vi "A提取产品ID.vi"(10 "字符串":string="B1_011308090450260075.280040.000090.00A000002600000020009999AA ") -> (3 "产品ID":string)   [LabVIEW 2013]
uses:
  <vilib>/Utility/error.llb/whitespace.ctl
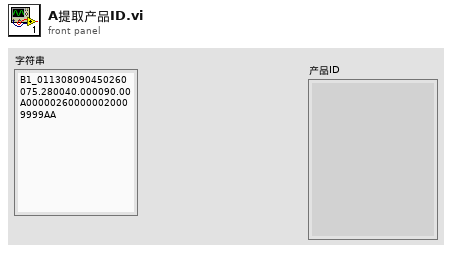
[diagram p1: front panel]
types:
  T1 = typedef "whitespace.ctl" = u16
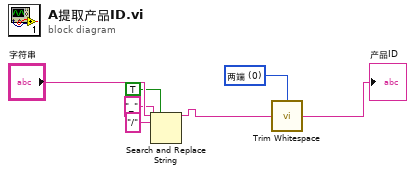
[diagram p0: block diagram]
diagram:
  w1 = T1 0 items=["两端", "字符串首端", "字符串末端"] ("location (both)")
  n1 = Search and Replace String(replace all?=TRUE ("替换全部？(F)"), input string="字符串", search string="/" ("搜索字符串"), replace string="_" ("替换字符串(\"\")")) -> (result string=w3:string)  [unwired: 4 in, 3 out]
  n2 = call <vilib>:"Trim Whitespace.vi"("string"=w3, "location (both)"=w1) -> ("trimmed string"=→"产品ID":string)
